vi "AO_mini_stageLaserControl.vi"() -> ()   [LabVIEW 2018]
uses:
  Drivers and controls/ASI/ASI_VIs/ASI Library/Shared_Serial/Axis Name.ctl
panel:
  out "Numeric status 2":dbl
  out "Response:":string
  in  "Send":bool
  in  "Command":string="W X"
  out "Position (um)":dbl[](array[numeric])=[0.0, 0.0, 0.0, -92.0, nan, nan] format="%#.1f"
  in  "Axis":T1[](array[typedef])=[enum."X", enum."Y", enum."Z", enum."Z", enum."F", enum."V"]
  in  "Get Position":bool
  out "Numeric status":dbl
  in  "Flip Mirror":sgl(ring) items=["EMCCD Camera"=0, "Wavefront sensor"=5]
  in  "flip mirror button":bool
  in  "2p shutter":refnum<k7>(container)
  in  "488 shutter":refnum<k7>(container)
  in  "stop":bool
  in  "VISA Stage":refnum<visa-resource-name>="COM5"
  in  "Z step":dbl=1.0
  in  "up":bool
  in  "down":bool
  in  "XY step":dbl=1.0
  in  "back":bool
  in  "front":bool
  in  "left":bool
  in  "right":bool
  # "Button defined by camera coordinates"
  # "WFS no tilt: X502, Y520 @EMCCD"
  # "Sample Stage"
  # "WF switch"
  # "Click to switch mirror position"
  # "x: +"
  # "z: +"
  # "Old Control (disabled)"
  # "y: -"
  # "1um = 10"
  # "EMCCD: 0"
  # "Wavefront Sensor: 5"
  # "Laser Shutter"
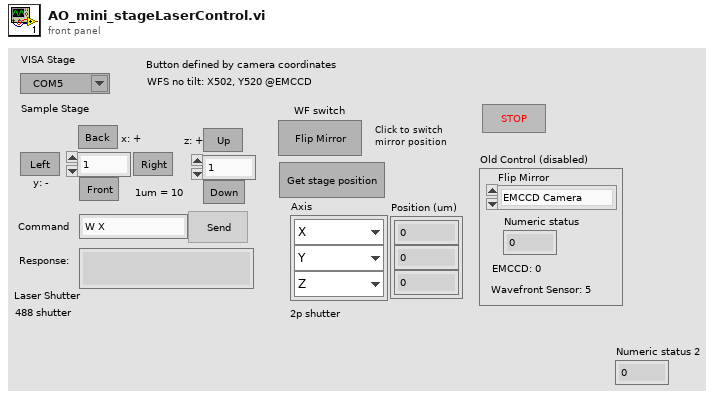
[diagram p1: front panel]
types:
  T1 = typedef "Axis Name.ctl" = enum8{"undefined", "A", "B", "C", "D", "E", "F", "G", "H", "I", "J", "K", "L", "M", "N", "O", "P", "Q", "R", "S", "T", "U", "V", "W", "X", "Y", "Z"}
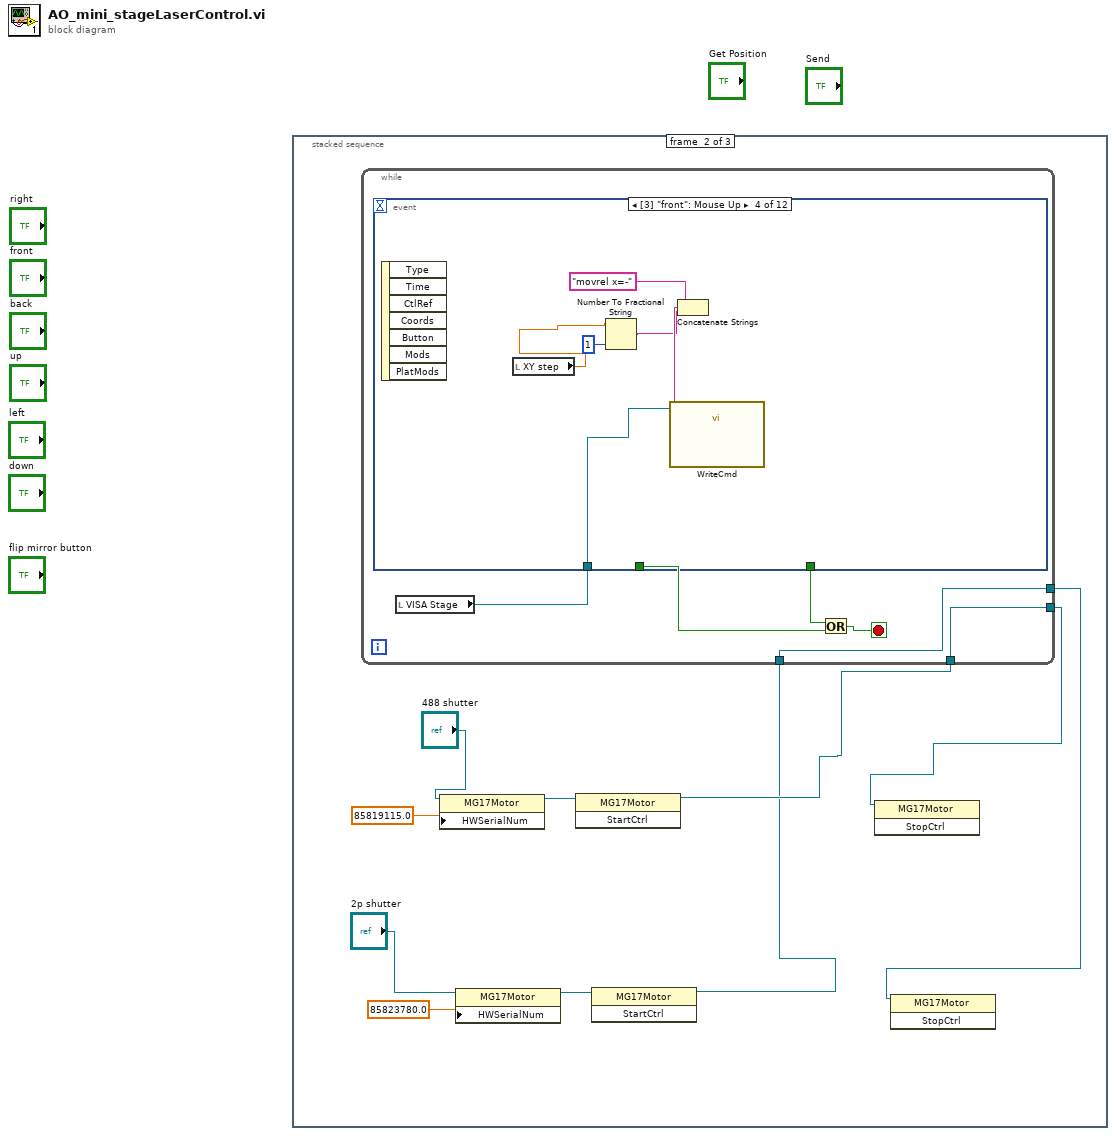
[diagram p0: block diagram]
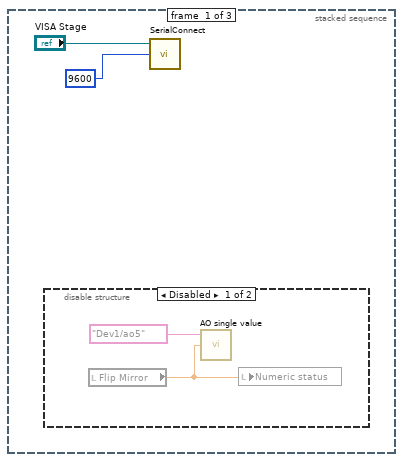
[diagram p2: hidden frame]
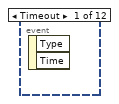
[diagram p4: hidden frame]
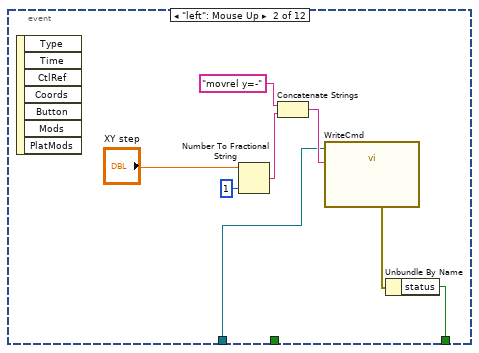
[diagram p5: hidden frame]
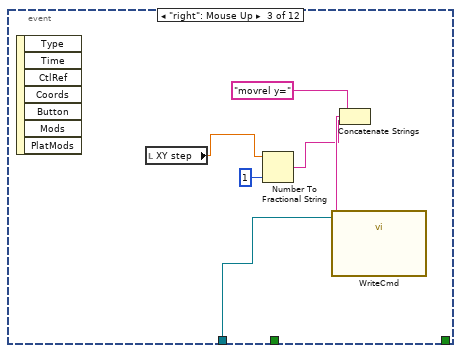
[diagram p6: hidden frame]
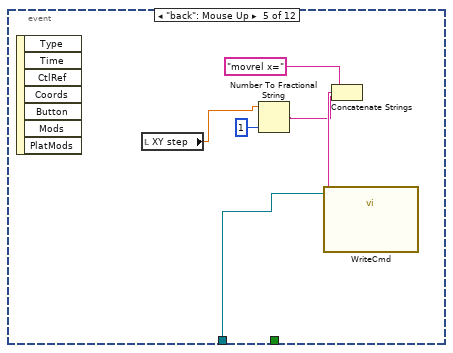
[diagram p7: hidden frame]
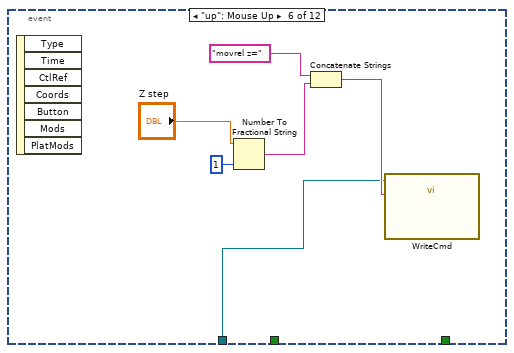
[diagram p8: hidden frame]
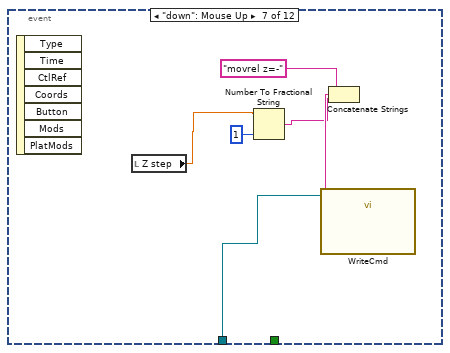
[diagram p9: hidden frame]
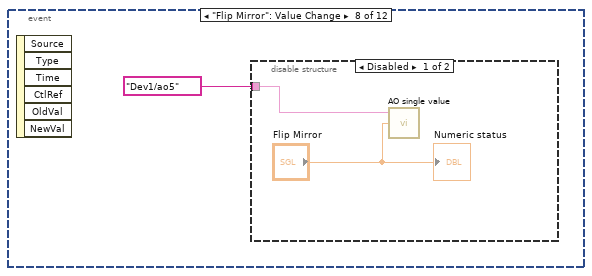
[diagram p10: hidden frame]
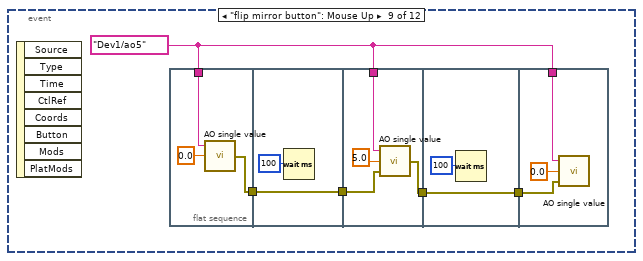
[diagram p12: hidden frame]
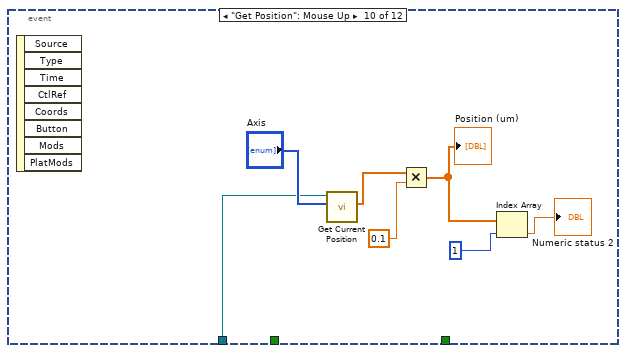
[diagram p13: hidden frame]
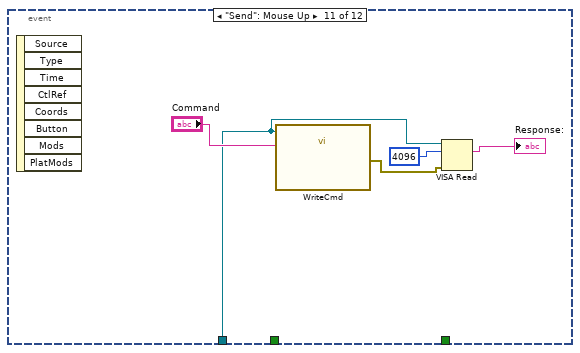
[diagram p14: hidden frame]
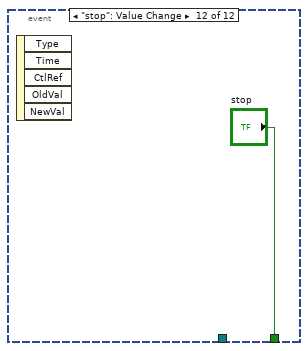
[diagram p15: hidden frame]
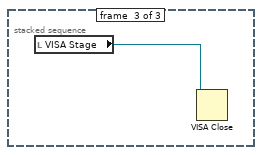
[diagram p16: hidden frame]
diagram:
  n1 = stacked-sequence {
    frame #0 {
      n2 = disable-structure shown="Disabled" {
        frame Disabled {
          n3 = local read "Flip Mirror"() -> (w3:sgl)
          n4 = call "AO single value.vi"("data"=w3, "physical channels"=tag "Dev1/ao5") -> ()  [unwired: 1 in, 1 out]
          n5 = local write "Numeric status"(w3) -> ()
        }
        frame Enabled {
        }
      }
      n6 = call "SerialConnect.vi"("baud rate (9600)"=9600, "VISA resource name"="VISA Stage") -> ()  [unwired: 1 in, 3 out]
    }
    frame #1 {
      n7 = property class="MG17Motor"(reference="488 shutter", "HWSerialNum"=85819115.0) -> (reference out=w14:refnum<k7>)  [unwired: 1 in, 1 out]
      n8 = property class="MG17Motor"(reference="2p shutter", "HWSerialNum"=85823780.0) -> (reference out=w9:refnum<k7>)  [unwired: 1 in, 1 out]
      n9 = invoke class="MG17Motor" method="StartCtrl"(reference=w14) -> (reference out=w13:refnum<k7>)  [unwired: 2 in, 2 out]
      n10 = invoke class="MG17Motor" method="StartCtrl"(reference=w9) -> (reference out=w6:refnum<k7>)  [unwired: 2 in, 2 out]
      n11 = while {
        tunnel: w13 -> [w17]
        tunnel: [w17] -> w12
        tunnel: w6 -> [w16]
        tunnel: [w16] -> w5
        stop <- w20 stop-if-true
        n12 = local read "VISA Stage"() -> (w15:refnum<visa-resource-name>)
        n13 = event shown="[3] \"front\": Mouse Up" {
          selector: _ -> [_ _ _ _ _ _ _ _ _ _ _ _]
          dyn-events: _ -> [_ _ _ _ _ _ _ _ _ _ _ _]
          timeout: _ -> [_ _ _ _ _ _ _ _ _ _ _ _]
          tunnel: [_ _ _ _ _ _ _ _ _ _ _ "stop"] -> w19
          tunnel: [_ w25 _ _ _ _ _ _ _ _ _ _] -> w18
          tunnel: w15 -> [_ w21 w29 w35 w41 w47 w53 _ _ w86 w91 _]
          event Timeout {
            n14 = event-data() -> ()  [unwired: 1 in, 2 out]
          }
          event "left": Mouse Up {
            n15 = event-data() -> ()  [unwired: 1 in, 7 out]
            n16 = Number To Fractional String(number="XY step", precision (6)=1) -> (F-format string=w22:string)  [unwired: 2 in]
            n17 = Concatenate Strings("movrel y=-", w22) -> (w27:string)
            n18 = call "WriteCmd.vi"("Command"=w27, "VISA resource name"=w21) -> ("error"=w26:errorcluster)  [unwired: 1 in, 1 out]
            n19 = Unbundle By Name(w26) -> ("status"=w25:bool)
          }
          event "right": Mouse Up {
            n20 = event-data() -> ()  [unwired: 1 in, 7 out]
            n21 = local read "XY step"() -> (w30:dbl)
            n22 = Number To Fractional String(number=w30, precision (6)=1) -> (F-format string=w31:string)  [unwired: 2 in]
            n23 = Concatenate Strings("movrel y=", w31) -> (w33:string)
            n24 = call "WriteCmd.vi"("Command"=w33, "VISA resource name"=w29) -> ()  [unwired: 1 in, 2 out]
          }
          event "front": Mouse Up {
            n25 = event-data() -> ()  [unwired: 1 in, 7 out]
            n26 = local read "XY step"() -> (w36:dbl)
            n27 = Number To Fractional String(number=w36, precision (6)=1) -> (F-format string=w37:string)  [unwired: 2 in]
            n28 = Concatenate Strings("movrel x=-", w37) -> (w39:string)
            n29 = call "WriteCmd.vi"("Command"=w39, "VISA resource name"=w35) -> ()  [unwired: 1 in, 2 out]
          }
          event "back": Mouse Up {
            n30 = event-data() -> ()  [unwired: 1 in, 7 out]
            n31 = local read "XY step"() -> (w42:dbl)
            n32 = Number To Fractional String(number=w42, precision (6)=1) -> (F-format string=w43:string)  [unwired: 2 in]
            n33 = Concatenate Strings("movrel x=", w43) -> (w45:string)
            n34 = call "WriteCmd.vi"("Command"=w45, "VISA resource name"=w41) -> ()  [unwired: 1 in, 2 out]
          }
          event "up": Mouse Up {
            n35 = event-data() -> ()  [unwired: 1 in, 7 out]
            n36 = Number To Fractional String(number="Z step", precision (6)=1) -> (F-format string=w50:string)  [unwired: 2 in]
            n37 = Concatenate Strings("movrel z=", w50) -> (w51:string)
            n38 = call "WriteCmd.vi"("Command"=w51, "VISA resource name"=w47) -> ()  [unwired: 1 in, 2 out]
          }
          event "down": Mouse Up {
            n39 = event-data() -> ()  [unwired: 1 in, 7 out]
            n40 = local read "Z step"() -> (w54:dbl)
            n41 = Number To Fractional String(number=w54, precision (6)=1) -> (F-format string=w55:string)  [unwired: 2 in]
            n42 = Concatenate Strings("movrel z=-", w55) -> (w57:string)
            n43 = call "WriteCmd.vi"("Command"=w57, "VISA resource name"=w53) -> ()  [unwired: 1 in, 2 out]
          }
          event "Flip Mirror": Value Change {
            n44 = event-data() -> ()  [unwired: 1 in, 6 out]
            n45 = disable-structure shown="Disabled" {
              disable-tunnel: tag "Dev1/ao5" ("physical channels") -> [w60 _]
              frame Disabled {
                n46 = call "AO single value.vi"("data"="Flip Mirror", "physical channels"=w60) -> ()  [unwired: 1 in, 1 out]
                "Numeric status" <- "Flip Mirror"
              }
              frame Enabled {
              }
            }
          }
          event "flip mirror button": Mouse Up {
            w62 = tag "Dev1/ao5" ("physical channels")
            n47 = event-data() -> ()  [unwired: 1 in, 8 out]
            n48 = flat-sequence {
              tunnel: [w69] -> w65
              tunnel: w62 -> [w67]
              tunnel: [w70] -> w66
              tunnel: w65 -> [w70]
              tunnel: w66 -> [w74]
              tunnel: [w73] -> w63
              tunnel: w62 -> [w72]
              tunnel: [w76] -> w64
              tunnel: w63 -> [w76]
              tunnel: w64 -> [w79]
              tunnel: w62 -> [w78]
              frame #0 {
                n49 = call "AO single value.vi"("data"=0.0, "physical channels"=w67) -> ("error out"=w69:errorcluster)  [unwired: 1 in]
              }
              frame #1 {
                n50 = Wait (ms)(milliseconds to wait=u32 100) -> ()  [unwired: 1 out]
              }
              frame #2 {
                n51 = call "AO single value.vi"("error in"=w74, "data"=5.0, "physical channels"=w72) -> ("error out"=w73:errorcluster)
              }
              frame #3 {
                n52 = Wait (ms)(milliseconds to wait=u32 100) -> ()  [unwired: 1 out]
              }
              frame #4 {
                n53 = call "AO single value.vi"("error in"=w79, "data"=0.0, "physical channels"=w78) -> ()  [unwired: 1 out]
              }
            }
          }
          event "Get Position": Mouse Up {
            n54 = event-data() -> ()  [unwired: 1 in, 8 out]
            n55 = call "Get Current Position.vi"("Array of axes"="Axis", "VISA in"=w86) -> ("Array of positions [internal units]"=w84:dbl[])  [unwired: 7 in, 2 out]
            n56 = Multiply(x=w84, y=0.1) -> (x*y=w83:dbl[])
            "Position (um)" <- w83
            n57 = Index Array(array=w83, index=1) -> (element=→"Numeric status 2":dbl)
          }
          event "Send": Mouse Up {
            n58 = event-data() -> ()  [unwired: 1 in, 8 out]
            n59 = call "WriteCmd.vi"("Command"="Command", "VISA resource name"=w91) -> ("error"=w89:errorcluster)  [unwired: 1 in, 1 out]
            n60 = VISA Read(VISA resource name=w91, byte count=u32 4096, error in (no error)=w89) -> (read buffer=→"Response:":string)  [unwired: 3 out]
          }
          event "stop": Value Change {
            n61 = event-data() -> ()  [unwired: 1 in, 5 out]
          }
        }
        n62 = Or(x=w18, y=w19) -> (x .or. y?=w20:bool)
      }
      n63 = invoke class="MG17Motor" method="StopCtrl"(reference=w12) -> ()  [unwired: 2 in, 3 out]
      n64 = invoke class="MG17Motor" method="StopCtrl"(reference=w5) -> ()  [unwired: 2 in, 3 out]
    }
    frame #2 {
      n65 = local read "VISA Stage"() -> (w94:refnum<visa-resource-name>)
      n66 = VISA Close(VISA resource name=w94) -> ()  [unwired: 1 in, 1 out]
    }
  }
